vi "write_agilent.vi"(3 "error in":errorcluster, 4 "data":string="func puls\nfreq 10\npuls:widt 0.001\nVolt 4\nvolt:offs 2\noutp on", 5 "address string":string="11") -> (0 "error out":errorcluster)   [LabVIEW 2013]
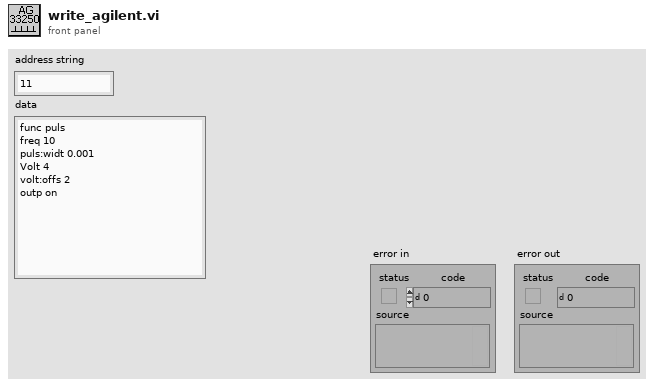
[diagram p1: front panel]
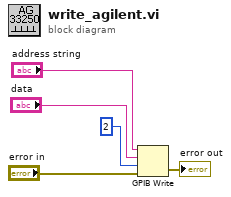
[diagram p0: block diagram]
diagram:
  n1 = GPIB Write(0:"address string", 1:"data", 2:2, 3:"error in") -> (6:→"error out":errorcluster)  [unwired: 1 in, 1 out]
